vi "subRegist_AddInfoIntoText.vi"(7 "log path":path, 11 "info to be added":string) -> ()   [LabVIEW 2015]
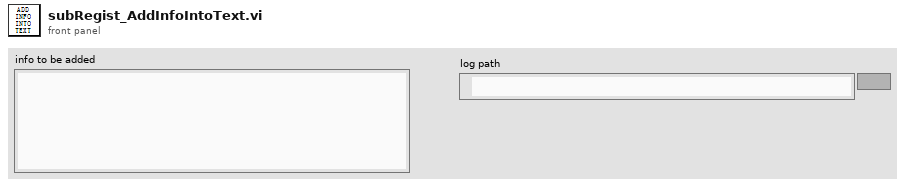
[diagram p1: front panel]
types:
  T1 = enum16{"open", "replace", "create", "open or create", "replace or create", "replace or create with confirmation"}
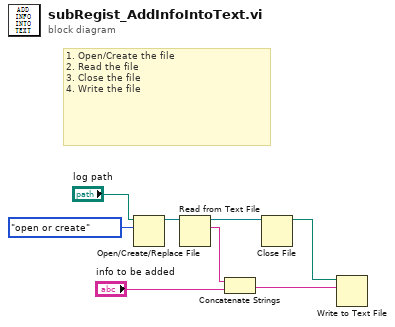
[diagram p0: block diagram]
diagram:
  # "1. Open/Create the file \n2. Read the file \n3. Close the file \n4. Write the file"
  n1 = Open/Create/Replace File(file path (use dialog)="log path", operation (0:open)=T1."open or create") -> (refnum out=w5:refnum<file>)  [unwired: 4 in, 2 out]
  n2 = Read from Text File(file (use dialog)=w5) -> (refnum out=w3:refnum<file>, text=w8:string)  [unwired: 3 in, 2 out]
  n3 = Concatenate Strings(w8, "info to be added") -> (w2:string)
  n4 = Close File(refnum=w3) -> (path=w1:path)  [unwired: 1 in, 1 out]
  n5 = Write to Text File(file (use dialog)=w1, text=w2) -> ()  [unwired: 2 in, 3 out]
